vi "_TangoReadUShortImageAttribute.vi"(3 "error in":errorcluster, 4 "attribute name":string, 5 "device name":string) -> (0 "error out":errorcluster, 1 "setpoint":u16[][](array[numeric]), 2 "value":u16[][](array[numeric]))   [LabVIEW 2014, in "tango.lvlib"]
uses:
  tango.lvlib
  Common VIs/Typedefs/_AttributeDataType_t.ctl
  Extractors/base/toUShortImage.vi
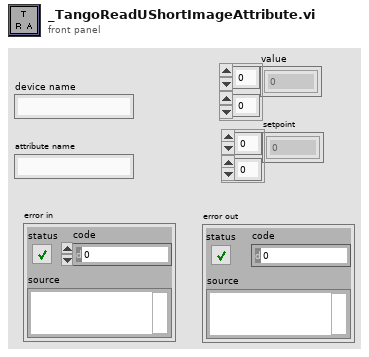
[diagram p1: front panel]
types:
  T1 = typedef "tango.lvlib/_AttributeDataType_t.ctl" = enum16{"STATE_SCA", "STATE_SPE", "STATE_IMG", "STRING_SCA", "STRING_SPE", "STRING_IMG", "BOOL_SCA", "BOOL_SPE", "BOOL_IMG", "UCHAR_SCA", "UCHAR_SPE", "UCHAR_IMG", "SHORT_SCA", "SHORT_SPE", "SHORT_IMG", "USHORT_SCA", "USHORT_SPE", "USHORT_IMG", "LONG_SCA", "LONG_SPE", "LONG_IMG", "ULONG_SCA", "ULONG_SPE", "ULONG_IMG", "LONG64_SCA", "LONG64_SPE", "LONG64_IMG", "ULONG64_SCA", "ULONG64_SPE", "ULONG64_IMG", "FLOAT_SCA", "FLOAT_SPE", "FLOAT_IMG", "DOUBLE_SCA", "DOUBLE_SPE", "DOUBLE_IMG", "UNKNOWN_DATA_TYPE"}
  T2 = typedef "tango.lvlib/_AttributeQuality_t.ctl" = enum16{"VALID", "INVALID", "ALARM", "CHANGING", "UNKNOWN_QUALITY"}
  T3 = cluster{"device name":string, "attribute name":string, "quality value":T2, "quality string":string, "timestamp":dbl, "dim. x":i32, "dim. y":i32, "value":u8[], "error code":i32, "error stack":string[], "data type":T1}[]
  T4 = cluster{"device name":string, "attribute name":string, "quality value":T2, "quality string":string, "timestamp":dbl, "dim. x":i32, "dim. y":i32, "value":u8[], "error code":i32, "error stack":string[], "data type":T1}
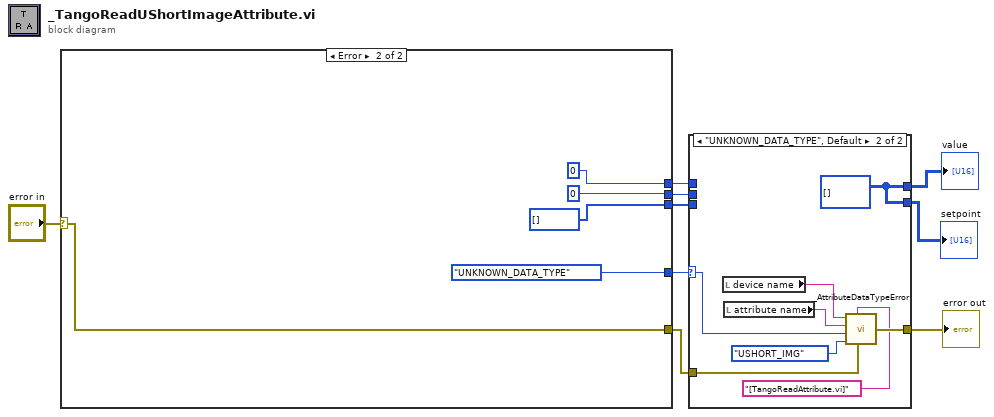
[diagram p0: block diagram]
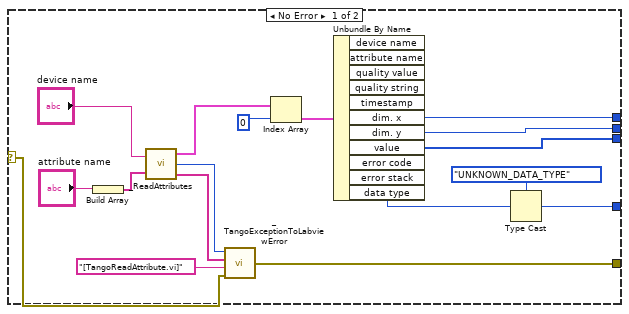
[diagram p2: hidden frame]
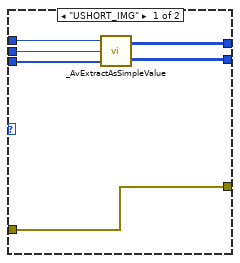
[diagram p3: hidden frame]
diagram:
  n1 = case shown="Error" "error in" {
    selector: "error in" -> [w10 w31]
    tunnel: [w15 _AttributeDataType_t."UNKNOWN_DATA_TYPE" ("Control")] -> w9
    tunnel: [w14 0 ("dim. x")] -> w8
    tunnel: [w13 0 ("dim. y")] -> w7
    tunnel: [w12 u8[] [] ("value")] -> w6
    tunnel: [w11 w31] -> w2
    frame No Error {
      n2 = Build Array("attribute name") -> (w21:string[])
      n3 = call "_ReadAttributes.vi"("device name"="device name", "attribute names"=w21) -> ("attribute values"=w23:T3, "error code"=w16:i32, "error stack"=w17:string[])
      n4 = call "_TangoExceptionToLabviewError.vi"("error in"=w10, "location"="[TangoReadAttribute.vi]", "error stack"=w17, "error code"=w16) -> ("error out"=w11:errorcluster)
      n5 = Index Array(array=w23, index=0 ("indice")) -> (element=w24:T4)
      n6 = Unbundle By Name(w24) -> ("dim. x"=w14:i32, "dim. y"=w13:i32, "value"=w12:u8[], "data type"=w19:T1)  [unwired: 7 out]
      n7 = Type Cast(type=_AttributeDataType_t."UNKNOWN_DATA_TYPE" ("Control"), x=w19) -> (*(type *) &x=w15:T1)
    }
    frame Error {
    }
  }
  n8 = case shown="\"UNKNOWN_DATA_TYPE\", Default" w9 {
    selector: w9 -> [_ w43]
    tunnel: w8 -> [w37 _]
    tunnel: w7 -> [w36 _]
    tunnel: w6 -> [w35 _]
    tunnel: [w34 w45] -> w4
    tunnel: [w33 w45] -> w3
    tunnel: w2 -> [w32 w39]
    tunnel: [w32 w44] -> w1
    frame "USHORT_IMG" {
      n9 = call-poly "_AvExtractAsSimpleValue.vi"("value_in"=w35, "dim_y"=w36, "dim_x"=w37) -> ("setpoint"=w33:u16[][], "value_out"=w34:u16[][])
    }
    frame "UNKNOWN_DATA_TYPE", Default {
      w45 = u16[][] [] ("value_out")
      n10 = local read "device name"() -> (w40:string)
      n11 = local read "attribute name"() -> (w41:string)
      n12 = call "_AttributeDataTypeError.vi"("error in"=w39, "location"="[TangoReadAttribute.vi]", "user Data Type"=_AttributeDataType_t."USHORT_IMG" ("Control"), "actual Data Type"=w43, "attribute name"=w41, "device name"=w40) -> ("error out"=w44:errorcluster)
    }
  }
  "error out" <- w1
  "value" <- w4
  "setpoint" <- w3
